vi "Broadcast Child Node Notifiers.vi"(8 "error in (no error)":errorcluster, 10 "Notification In":variant, 11 "Root Actor in":refnum<class "Root Actor.lvclass">) -> (0 "error out":errorcluster, 3 "Root Actor out":refnum<class "Root Actor.lvclass">)   [LabVIEW 2024, in "Root Actor.lvclass"]
uses:
  Root Actor.lvclass
  Root Actor.lvclass/Root Actor.ctl
  Notifier Controller/Notifier Controller.lvclass
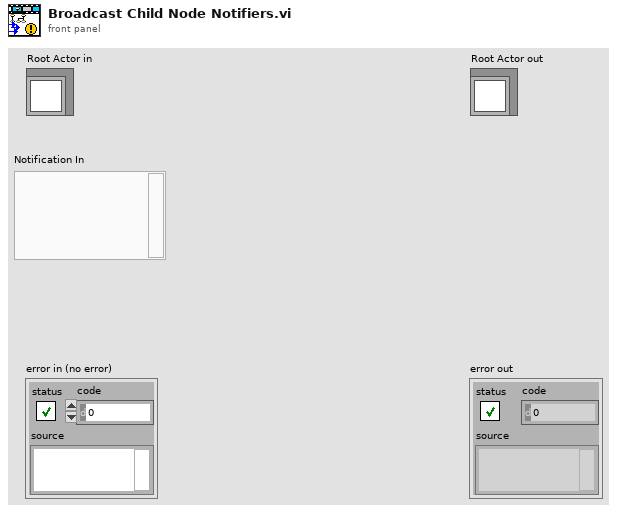
[diagram p1: front panel]
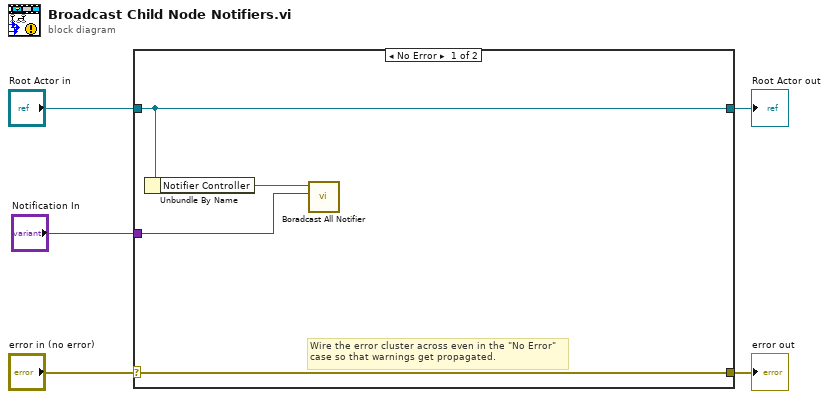
[diagram p0: block diagram]
diagram:
  n1 = case shown="No Error" "error in (no error)" {
    selector: "error in (no error)" -> [w9 w11]
    tunnel: [w9 w11] -> w4
    tunnel: [w8 w10] -> w2
    tunnel: "Root Actor in" -> [w8 w10]
    tunnel: "Notification In" -> [w6 _]
    frame No Error {
      # "Wire the error cluster across even in the \"No Error\"\ncase so that warnings get propagated."
      n2 = Unbundle By Name(w8) -> ("Notifier Controller"=w7:refnum<class "Notifier Controller.lvclass">)
      n3 = call-dynamic "Boradcast All Notifier.vi"("Notification In"=w6, "Notifier Controller in"=w7) -> ()  [unwired: 8 in, 2 out]
    }
    frame Error {
    }
  }
  "error out" <- w4
  "Root Actor out" <- w2
